vi "settings-recall-mag-actuator.vi"() -> (0 "error out":errorcluster, 3 "mag-settings":T1={"COM Port (COM10)"="COM10", "ADAM-ID"=1.0, "ADAM-DO-channel"=1.0, "Period (Seconds)"=5.0, "Duty Cycle"=10.0, "Eng Mode"=TRUE}, 5 "Settings Recalled":bool)   [LabVIEW 2021]
uses:
  mag-settings.ctl
  <vilib>/Utility/config.llb/Read Key (String).vi
  <vilib>/Utility/config.llb/Read Key (Double).vi
  <vilib>/Utility/config.llb/Read Key (Boolean).vi
  <vilib>/Utility/config.llb/NI_LVConfig.lvlib
panel:
  out "config.ini Found":bool
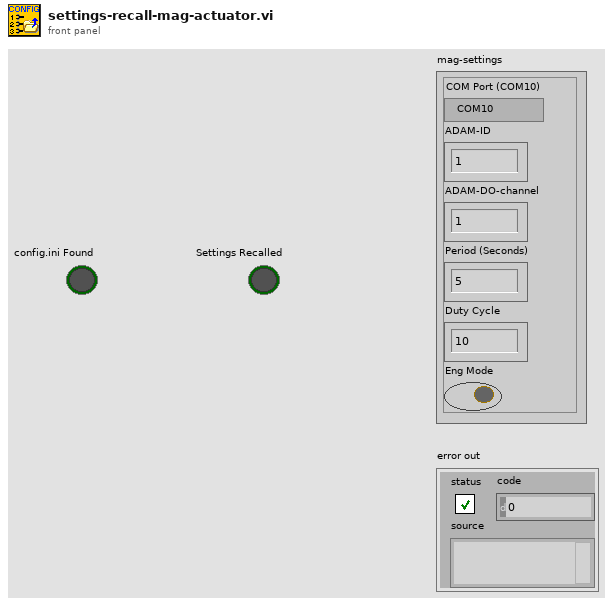
[diagram p1: front panel]
types:
  T1 = typedef "mag-settings.ctl" = cluster{"COM Port (COM10)":refnum<visa-resource-name>, "ADAM-ID":dbl, "ADAM-DO-channel":dbl, "Period (Seconds)":dbl, "Duty Cycle":dbl, "Eng Mode":bool}
  T2 = enum16{"open", "replace", "create", "open or create", "replace or create", "replace or create with confirmation"}
  T3 = typedef "NI_LVConfig.lvlib/Config Data RefNum.ctl" = refnum<k1>
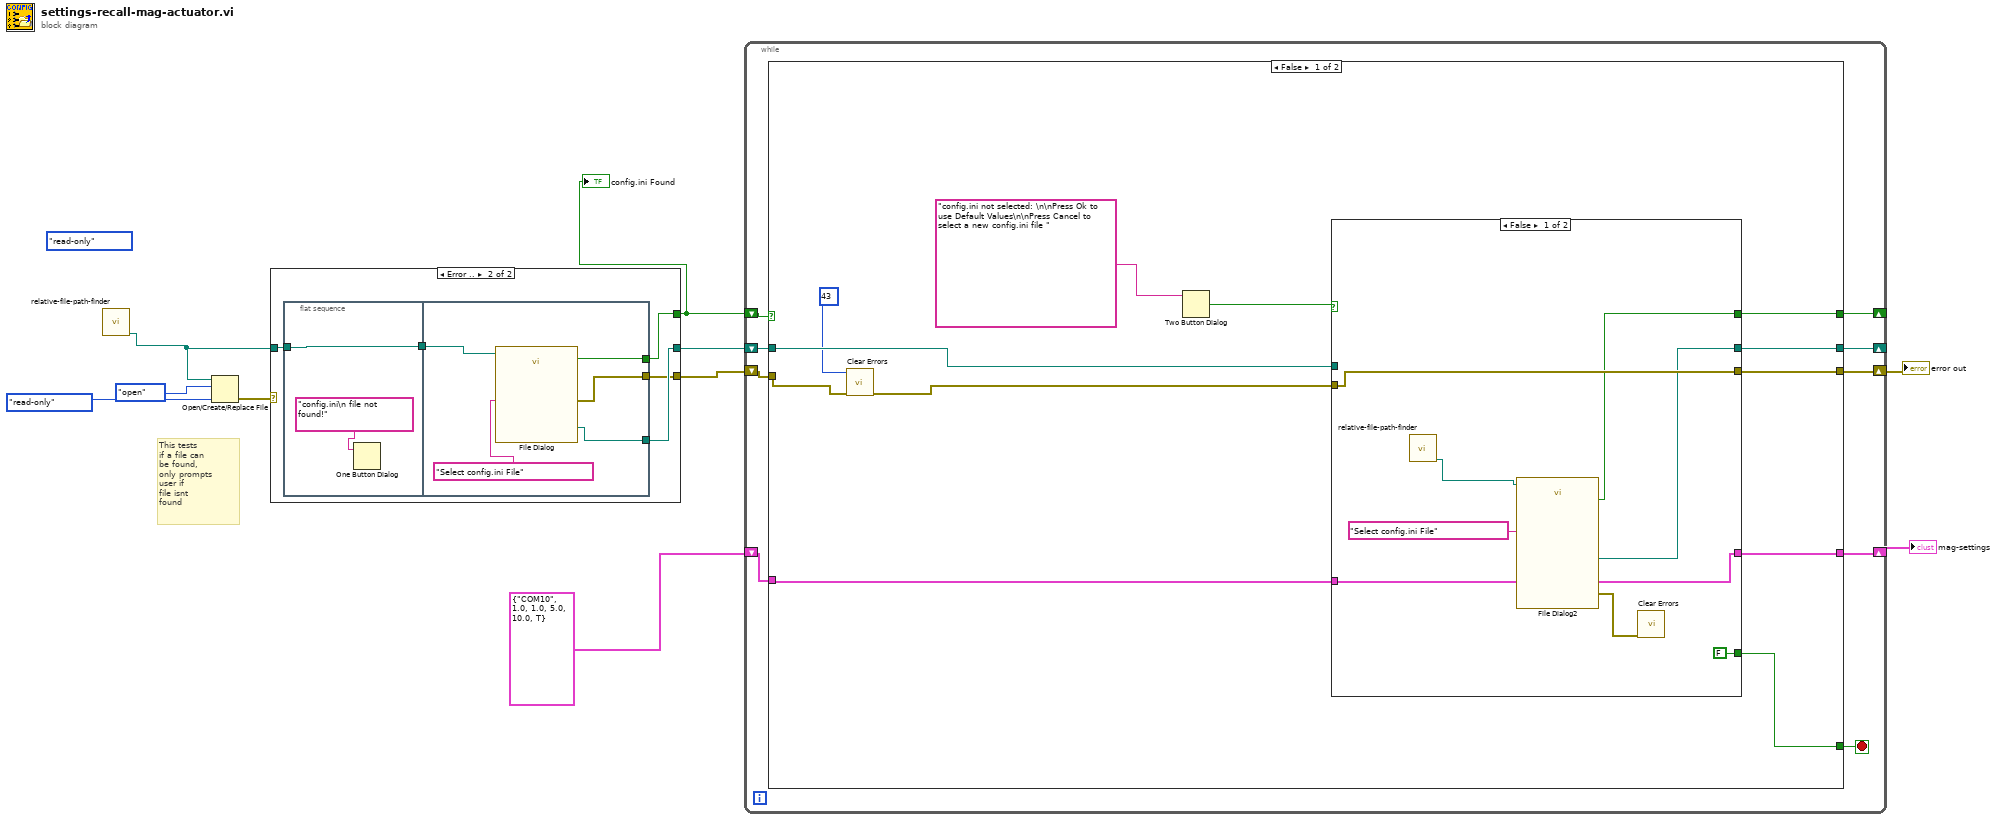
[diagram p0: block diagram]
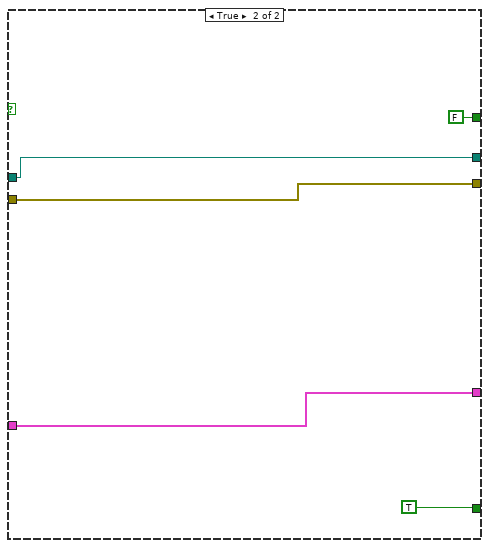
[diagram p2: hidden frame]
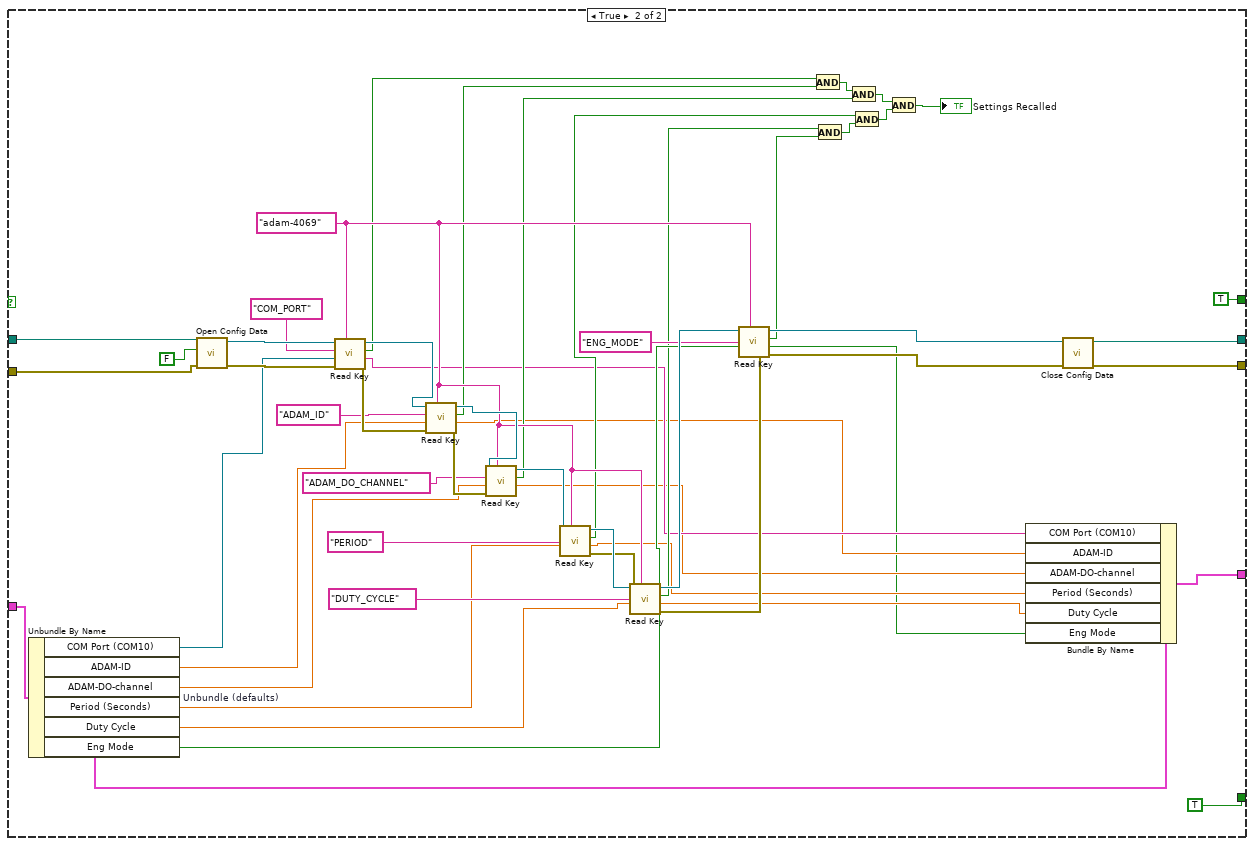
[diagram p3: hidden frame]
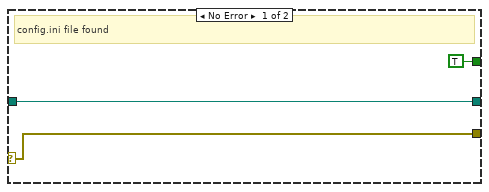
[diagram p4: hidden frame]
diagram:
  (unwired) enum16{"read/write", "read-only", "write-only"}."read-only" ("access (0:read/write)")
  # "This tests\nif a file can\nbe found,\nonly prompts\nuser if\nfile isnt\nfound"
  n1 = call "relative-file-path-finder.vi"() -> ("Config File"=w5:path)  [unwired: 8 in, 3 out]
  n2 = Open/Create/Replace File(file path (use dialog)=w5, operation (0:open)=T2."open", access (0:read/write)=enum16{"read/write", "read-only", "write-only"}."read-only") -> (error out=w6:errorcluster)  [unwired: 3 in, 2 out]
  n3 = case shown="Error .." w6 {
    selector: w6 -> [w11 _]
    tunnel: w5 -> [w13 w16]
    tunnel: [w13 w18] -> w4
    tunnel: [TRUE ("exists") w15] -> w1
    tunnel: [w11 w14] -> w3
    frame No Error {
      # "config.ini file found"
    }
    frame Error {
      n4 = flat-sequence {
        tunnel: [w19] -> w17
        tunnel: w16 -> [w19]
        tunnel: [w22] -> w18
        tunnel: [w25] -> w15
        tunnel: w17 -> [w23]
        tunnel: [w21] -> w14
        frame #0 {
          n5 = One Button Dialog(message="config.ini\n file not found!") -> ()  [unwired: 1 in, 1 out]
        }
        frame #1 {
          n6 = call "File Dialog"("start path"=w23, "prompt"="Select config.ini File") -> ("selected path"=w22:path, "exists"=w25:bool, "error out"=w21:errorcluster)  [unwired: 10 in, 1 out]
        }
      }
    }
  }
  "config.ini Found" <- w1
  n7 = while {
    shift-right: [w33] -> w9
    shift-left: T1 {"COM Port (COM10)"="COM10", "ADAM-ID"=1.0, "ADAM-DO-channel"=1.0, "Period (Seconds)"=5.0, "Duty Cycle"=10.0, "Eng Mode"=TRUE} ("mag-settings") -> [w34]
    shift-right: [w30] -> w2
    shift-left: w3 -> [w31]
    shift-right: [w27] -> _
    shift-left: w4 -> [w32]
    shift-right: [w26] -> _
    shift-left: w1 -> [w29]
    stop <- w28 stop-if-true
    n8 = case shown="False" w29 {
      tunnel: w34 -> [w43 w98]
      tunnel: [w44 w97] -> w33
      tunnel: w32 -> [w39 w65]
      tunnel: w31 -> [w36 w64]
      tunnel: [w42 w63] -> w30
      tunnel: [w41 TRUE] -> w28
      tunnel: [w40 w61] -> w27
      tunnel: [w38 TRUE ("exists")] -> w26
      frame False {
        n9 = call <vilib>:"Clear Errors.vi"("error in (no error)"=w36, "specific error code to clear (0: all)"=43) -> ("error out"=w35:errorcluster)  [unwired: 4 in, 1 out]
        n10 = Two Button Dialog(message="config.ini not selected: \n\nPress Ok to use Default Values\n\nPress Cancel to select a new config.ini file ") -> (T button?=w45:bool)  [unwired: 2 in]
        n11 = case shown="False" w45 {
          tunnel: [w50 w59] -> w44
          tunnel: w43 -> [w50 w59]
          tunnel: [w54 w58] -> w42
          tunnel: w35 -> [w54 w58]
          tunnel: [FALSE TRUE] -> w41
          tunnel: [w51 w56] -> w40
          tunnel: w39 -> [_ w56]
          tunnel: [w47 FALSE ("exists")] -> w38
          frame False {
            n12 = call "relative-file-path-finder.vi"() -> ("Config File"=w52:path)  [unwired: 8 in, 3 out]
            n13 = call "File Dialog2"("start path"=w52, "prompt"="Select config.ini File") -> ("selected path"=w51:path, "exists"=w47:bool, "error out"=w48:errorcluster)  [unwired: 10 in, 1 out]
            n14 = call <vilib>:"Clear Errors.vi"("error in (no error)"=w48) -> ()  [unwired: 5 in, 2 out]
          }
          frame True {
          }
        }
      }
      frame True {
        w87 = "adam-4069" ("section")
        n15 = Unbundle By Name "Unbundle (defaults)"(w98) -> ("COM Port (COM10)"=w108:refnum<visa-resource-name>, "ADAM-ID"=w82:dbl, "ADAM-DO-channel"=w83:dbl, "Period (Seconds)"=w84:dbl, "Duty Cycle"=w85:dbl, "Eng Mode"=w86:bool)
        n16 = call <vilib>:"Open Config Data.vi"("error in (no error)"=w64, "create file if necessary (T)"=FALSE, "configuration file path"=w65) -> ("error out"=w111:errorcluster, "refnum"=w110:T3)  [unwired: 6 in, 1 out]
        n17 = call-poly <vilib>:"Read Key.vi"("section"=w87, "error in (no error)"=w111, "default value"=w108, "key"="COM_PORT", "refnum"=w110) -> ("error out"=w92:errorcluster, "value"=w72:string, "found?"=w79:bool, "refnum out"=w93:T3)  [unwired: 3 in]
        n18 = call-poly <vilib>:"Read Key.vi"("section"=w87, "error in (no error)"=w92, "default value"=w82, "key"="ADAM_ID", "refnum"=w93) -> ("error out"=w90:errorcluster, "value"=w71:dbl, "found?"=w78:bool, "refnum out"=w91:T3)  [unwired: 3 in]
        n19 = call-poly <vilib>:"Read Key.vi"("section"=w87, "error in (no error)"=w90, "default value"=w83, "key"="ADAM_DO_CHANNEL", "refnum"=w91) -> ("value"=w70:dbl, "found?"=w76:bool, "refnum out"=w77:T3)  [unwired: 3 in, 1 out]
        n20 = call-poly <vilib>:"Read Key.vi"("section"=w87, "default value"=w84, "key"="PERIOD", "refnum"=w77) -> ("error out"=w104:errorcluster, "value"=w69:dbl, "found?"=w75:bool, "refnum out"=w106:T3)  [unwired: 4 in]
        n21 = call-poly <vilib>:"Read Key.vi"("section"=w87, "error in (no error)"=w104, "default value"=w85, "key"="DUTY_CYCLE", "refnum"=w106) -> ("error out"=w102:errorcluster, "value"=w68:dbl, "found?"=w74:bool, "refnum out"=w103:T3)  [unwired: 3 in]
        n22 = call-poly <vilib>:"Read Key.vi"("section"=w87, "error in (no error)"=w102, "default value"=w86, "key"="ENG_MODE", "refnum"=w103) -> ("error out"=w99:errorcluster, "value"=w67:bool, "found?"=w73:bool, "refnum out"=w100:T3)  [unwired: 3 in]
        n23 = And(x=w79, y=w78) -> (x .and. y?=w80:bool)
        n24 = And(x=w74, y=w73) -> (x .and. y?=w81:bool)
        n25 = And(x=w80, y=w76) -> (x .and. y?=w96:bool)
        n26 = And(x=w75, y=w81) -> (x .and. y?=w95:bool)
        n27 = And(x=w96, y=w95) -> (x .and. y?=→"Settings Recalled":bool)
        n28 = Bundle By Name(cluster=w98, "COM Port (COM10)"=w72, "ADAM-ID"=w71, "ADAM-DO-channel"=w70, "Period (Seconds)"=w69, "Duty Cycle"=w68, "Eng Mode"=w67) -> (w97:T1)
        n29 = call <vilib>:"Close Config Data.vi"("error in (no error)"=w99, "refnum"=w100) -> ("error out"=w63:errorcluster, "file path"=w61:path)  [unwired: 8 in]
      }
    }
  }
  "mag-settings" <- w9
  "error out" <- w2
